vi "to string 1.0.vi"(8 "error in (no error)":errorcluster, 10 "data in":string, 11 "E2E configuration in":refnum<class "E2E Tag Exchange configuration.lvclass">) -> (0 "error out":errorcluster, 2 "data out":string, 3 "E2E configuration out":refnum<class "E2E Tag Exchange configuration.lvclass">)   [LabVIEW 2015, in "E2E Tag Exchange configuration.lvclass"]
uses:
  E2E Tag Exchange configuration.lvclass
  E2E Tag Exchange configuration.lvclass/E2E Tag Exchange configuration.ctl
  <vilib>/NI/Tag Bus Module Framework/channel/TBM channel.lvclass
  <vilib>/NI/Configuration Framework/serializable configuration/NISE_CEF_serializable configuration.lvclass
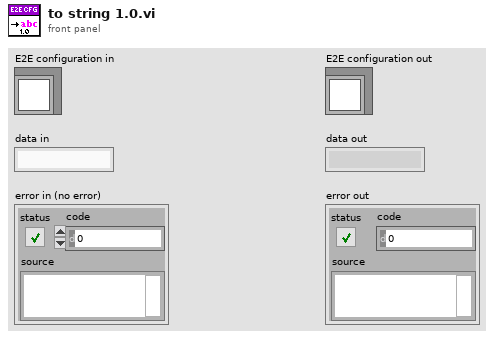
[diagram p1: front panel]
types:
  T1 = typedef "E2E Tag Exchange configuration.lvclass/Runtime Implementation.ctl" = enum16{"RT FIFO", "UDP"}
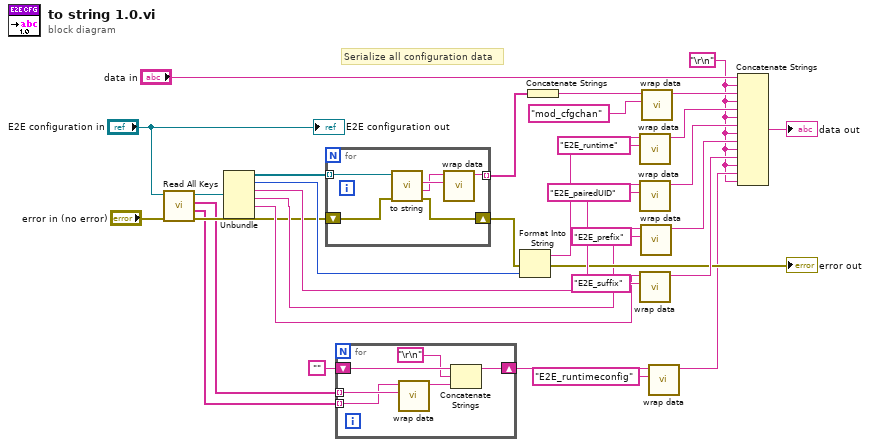
[diagram p0: block diagram]
diagram:
  w1 = "\r\n"
  # "Serialize all configuration data"
  n1 = call "Read All Keys.vi"("error in"="error in (no error)", "E2E configuration in"="E2E configuration in") -> ("error out"=w8:errorcluster, "Values"=w6:string[], "Keys"=w7:string[], "E2E configuration out"=w9:refnum<class "E2E Tag Exchange configuration.lvclass">)  [unwired: 6 in]
  n2 = Unbundle(w9) -> (w27:refnum<class "TBM channel.lvclass">[], w26:T1, w23:string, w13:string, w12:string)  [unwired: 1 out]
  n3 = for {
    tunnel: w27 -> [w35] mode=indexing
    tunnel: [w37] -> w28 mode=indexing
    shift-right: [w36] -> w25
    shift-left: w8 -> [w34]
    n4 = call-dynamic "to string.vi"("error in"=w34, "channel in"=w35) -> ("error out"=w36:errorcluster, "channel data"=w38:string, "identifier"=w39:string)  [unwired: 6 in, 1 out]
    n5 = call <vilib>:"wrap data.vi"("identifier"=w39, "data to wrap"=w38) -> ("wrapped data"=w37:string)  [unwired: 9 in]
  }
  n6 = for {
    tunnel: w7 -> [w45] mode=indexing
    tunnel: w6 -> [w44] mode=indexing
    shift-right: [w42] -> w4
    shift-left: "" -> [w41]
    n7 = call <vilib>:"wrap data.vi"("identifier"=w45, "data to wrap"=w44) -> ("wrapped data"=w43:string)  [unwired: 9 in]
    n8 = Concatenate Strings(w41, "\r\n", w43) -> (w42:string)
  }
  n9 = Format Into String(error in=w25, w26) -> (resulting string=w24:string, error out=→"error out":errorcluster)  [unwired: 2 in]
  n10 = Concatenate Strings(w28) -> (w29:string)
  n11 = call <vilib>:"wrap data.vi"("identifier"="E2E_runtime", "data to wrap"=w24) -> ("wrapped data"=w20:string)  [unwired: 9 in]
  n12 = call <vilib>:"wrap data.vi"("identifier"="E2E_pairedUID", "data to wrap"=w23) -> ("wrapped data"=w19:string)  [unwired: 9 in]
  n13 = call <vilib>:"wrap data.vi"("identifier"="E2E_suffix", "data to wrap"=w12) -> ("wrapped data"=w17:string)  [unwired: 9 in]
  n14 = call <vilib>:"wrap data.vi"("identifier"="E2E_prefix", "data to wrap"=w13) -> ("wrapped data"=w18:string)  [unwired: 9 in]
  n15 = call <vilib>:"wrap data.vi"("identifier"="mod_cfgchan", "data to wrap"=w29) -> ("wrapped data"=w32:string)  [unwired: 9 in]
  n16 = call <vilib>:"wrap data.vi"("identifier"="E2E_runtimeconfig", "data to wrap"=w4) -> ("wrapped data"=w2:string)  [unwired: 9 in]
  n17 = Concatenate Strings("data in", w1, w32, w1, w20, w1, w19, w1, w18, w1, w17, w1, w2, w1) -> (→"data out":string)
  "E2E configuration out" <- "E2E configuration in"
